vi "master.vi"() -> ()   [LabVIEW 2017]
panel:
  in  "Number of Columns":i32
  in  "Path":string
  out "data":dynamicdata(graph)
  in  "Number of Rows":i32
  in  "Sampling Rate (Hz)":dbl=100.0
  in  "Number of Samples":i32=100
  in  "Pixel Size (mm)":string
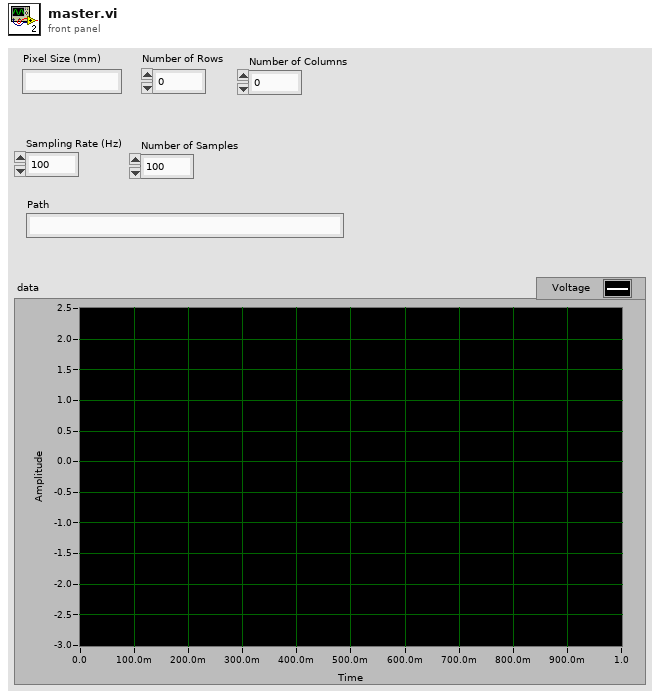
[diagram p1: front panel]
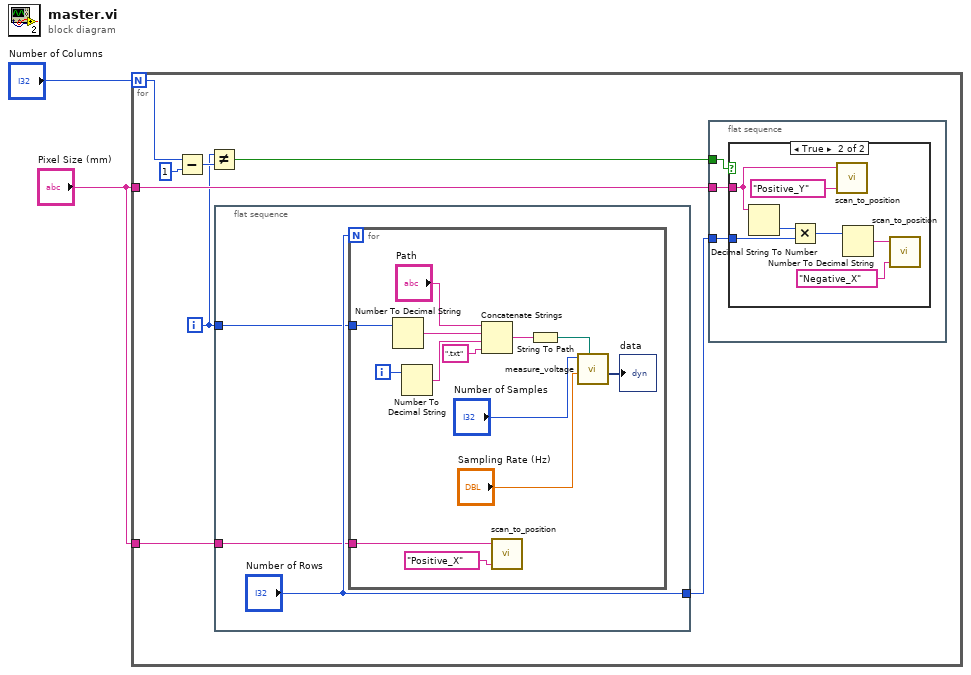
[diagram p0: block diagram]
diagram:
  n1 = for {
    N: "Number of Columns" -> [w4]
    tunnel: "Pixel Size (mm)" -> [w9]
    tunnel: "Pixel Size (mm)" -> [w8]
    i -> [w3]
    n2 = Subtract(x=w4, y=1) -> (x-y=w6:i32)
    n3 = Not Equal?(x=w3, y=w6) -> (x != y?=w5:bool)
    n4 = flat-sequence {
      tunnel: ["Number of Rows"] -> w10
      tunnel: w9 -> [w22]
      tunnel: w3 -> [w21]
      frame #0 {
        n5 = for {
          N: "Number of Rows" -> [_]
          tunnel: w22 -> [w33]
          tunnel: w21 -> [w28]
          i -> [w29]
          n6 = Number To Decimal String(number=w28) -> (decimal integer string=w32:string)  [unwired: 1 in]
          n7 = Number To Decimal String(number=w29) -> (decimal integer string=w31:string)  [unwired: 1 in]
          n8 = Concatenate Strings("Path", w32, w31, ".txt" ("string")) -> (w35:string)
          n9 = call "scan_to_position.vi"("Direction to Move"="Positive_X", "Pixel Size (mm)"=w33) -> ()  [unwired: 7 in]
          n10 = String To Path(string=w35) -> (path=w26:path)
          n11 = call "measure_voltage.vi"("Filename"=w26, "rate"="Sampling Rate (Hz)", "number of samples"="Number of Samples") -> ("data"=→"data":dynamicdata)  [unwired: 6 in]
        }
      }
    }
    n12 = flat-sequence {
      tunnel: w10 -> [w13]
      tunnel: w8 -> [w12]
      tunnel: w5 -> [w11]
      frame #0 {
        n13 = case shown="True" w11 {
          tunnel: w13 -> [_ w18]
          tunnel: w12 -> [_ w15]
          frame False {
          }
          frame True {
            n14 = Decimal String To Number(string=w15) -> (number=w19:i32)  [unwired: 2 in, 1 out]
            n15 = Multiply(x=w19, y=w18) -> (x*y=w17:i32)
            n16 = call "scan_to_position.vi"("Direction to Move"="Positive_Y", "Pixel Size (mm)"=w15) -> ()  [unwired: 7 in]
            n17 = Number To Decimal String(number=w17) -> (decimal integer string=w14:string)  [unwired: 1 in]
            n18 = call "scan_to_position.vi"("Direction to Move"="Negative_X", "Pixel Size (mm)"=w14) -> ()  [unwired: 7 in]
          }
        }
      }
    }
  }
